vi "DevB.Open Device.vi"(8 "error in (no error)":errorcluster, 10 "Port":refnum<visa-resource-name>) -> (0 "error out":errorcluster, 3 "DevB Session out":T1)   [LabVIEW 2018]
uses:
  typedefs/DevB.Session.ctl
  <vilib>/Instr/_visa.llb/VISA Configure Serial Port (Instr).vi
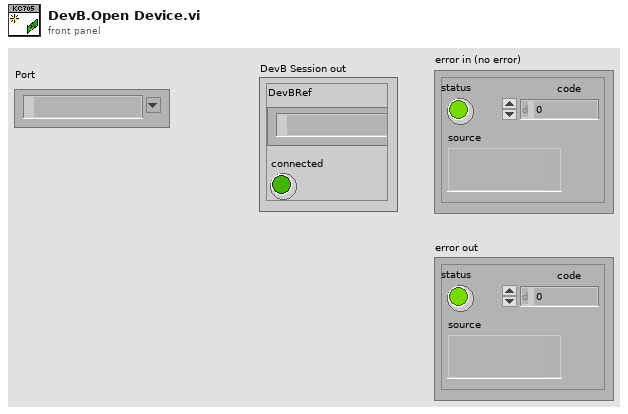
[diagram p1: front panel]
types:
  T1 = typedef "DevB.Session.ctl" = cluster{"DevBRef":refnum<visa-resource-name>, "connected":bool}
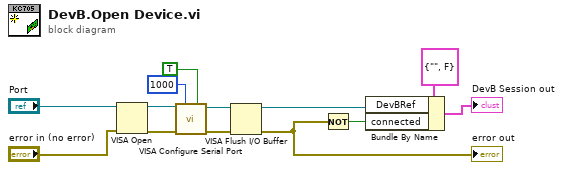
[diagram p0: block diagram]
diagram:
  n1 = VISA Open(error in (no error)="error in (no error)", VISA resource name="Port") -> (VISA resource name=w12:refnum<visa-resource-name>, error out=w11:errorcluster)  [unwired: 3 in]
  n2 = call-poly "VISA Configure Serial Port"("VISA resource name"=w12, "timeout (10sec)"=u32 1000, "Enable Termination\nChar (T)"=TRUE ("Enable Termination\nChar (T)"), "error in (no error)"=w11) -> ("VISA resource name out"=w5:refnum<visa-resource-name>, "error out"=w3:errorcluster)  [unwired: 10 in]
  n3 = VISA Flush I/O Buffer(VISA resource name=w5, error in (no error)=w3) -> (VISA resource name out=w4:refnum<visa-resource-name>, error out=w2:errorcluster)  [unwired: 1 in]
  "error out" <- w2
  n4 = Not(x=w2) -> (.not. x?=w1:bool)
  n5 = Bundle By Name(cluster=T1 {"DevBRef"="", "connected"=FALSE} ("DevB Session in"), "DevBRef"=w4, "connected"=w1) -> (→"DevB Session out":T1)
